vi "solar_voy_def Find Item (Name).vi"(9 "ITEM_NAME":string, 10 "ITEMS":T1[](array[typedef])) -> (2 "Index":i32)   [LabVIEW 2018]
doc: "This searches for an item by name."
uses:
  solar_voy_def_ctl ITEM TYPE.ctl
  type/solar_type Item Type.ctl
  solar_voy_def_ctl ITEM.ctl
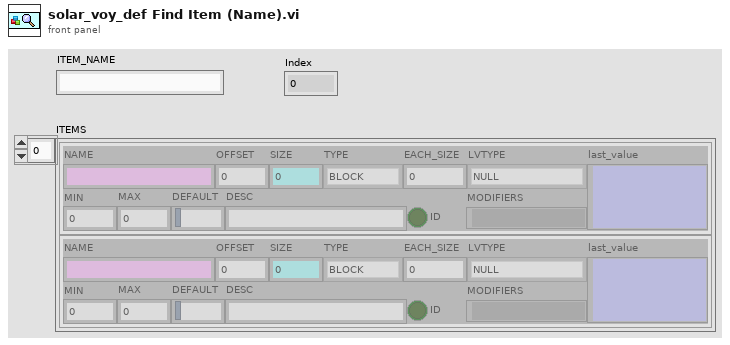
[diagram p1: front panel]
types:
  T1 = typedef "solar_voy_def_ctl ITEM.ctl" = cluster{"NAME":string, "OFFSET":i32, "SIZE":i32, "TYPE":T2, "EACH_SIZE":i32, "LVTYPE":T3, "MIN":dbl, "MAX":dbl, "DEFAULT":string, "DESC":string, "ID":bool, "MODIFIERS":variant, "last_value":variant}
  T2 = typedef "solar_voy_def_ctl ITEM TYPE.ctl" = enum8{"BLOCK", "INT", "UINT", "FLOAT", "STRING"}
  T3 = typedef "solar_type Item Type.ctl" = enum16{"NULL", "UNKNOWN", "CLUSTER", "I8", "I16", "I32", "I64", "U8", "U16", "U32", "U64", "U8_ENUM", "U16_ENUM", "U32_ENUM", "SGL", "DBL", "BOOLEAN", "STRING", "PATH", "VISA", "TAG", "TIME", "I8_1D", "I16_1D", "I32_1D", "I64_1D", "U8_1D", "U16_1D", "U32_1D", "U64_1D", "U8_ENUM_1D", "U16_ENUM_1D", "U32_ENUM_1D", "SGL_1D", "DBL_1D", "BOOLEAN_1D", "STRING_1D", "PATH_1D", "VISA_1D", "TAG_1D", "TIME_1D", "I8_2D", "I16_2D", "I32_2D", "I64_2D", "U8_2D", "U16_2D", "U32_2D", "U64_2D", "U8_ENUM_2D", "U16_ENUM_2D", "U32_ENUM_2D", "SGL_2D", "DBL_2D", "BOOLEAN_2D", "STRING_2D", "PATH_2D", "VISA_2D", "TAG_2D", "TIME_2D"}
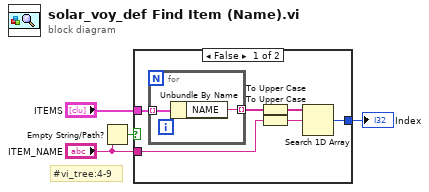
[diagram p0: block diagram]
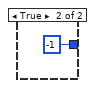
[diagram p2: hidden frame]
diagram:
  # "#vi_tree:4-9"
  n1 = Empty String/Path?(string/path="ITEM_NAME") -> (empty?=w1:bool)
  n2 = case shown="False" w1 {
    tunnel: "ITEMS" -> [w10 _]
    tunnel: "ITEM_NAME" -> [w6 _]
    tunnel: [w5 -1 ("index of element")] -> w3
    frame False {
      n3 = for {
        tunnel: w10 -> [w12] mode=indexing
        tunnel: [w11] -> w9 mode=indexing
        n4 = Unbundle By Name(w12) -> ("NAME"=w11:string)
      }
      n5 = To Upper Case(1:w9) -> (0:w8:string[])
      n6 = To Upper Case(1:w6) -> (0:w7:string)
      n7 = Search 1D Array(1D array=w8, element=w7) -> (index of element=w5:i32)  [unwired: 1 in]
    }
    frame True {
    }
  }
  "Index" <- w3
